vi "Destroy queues.vi"(8 "error in (no error)":errorcluster, 11 "Messenger in":refnum<class "Messenger.lvclass">) -> (0 "error out":errorcluster, 3 "Messenger out":refnum<class "Messenger.lvclass">)   [LabVIEW 2018, in "Messenger.lvclass"]
uses:
  Messenger.lvclass
  Messenger.lvclass/Messenger.ctl
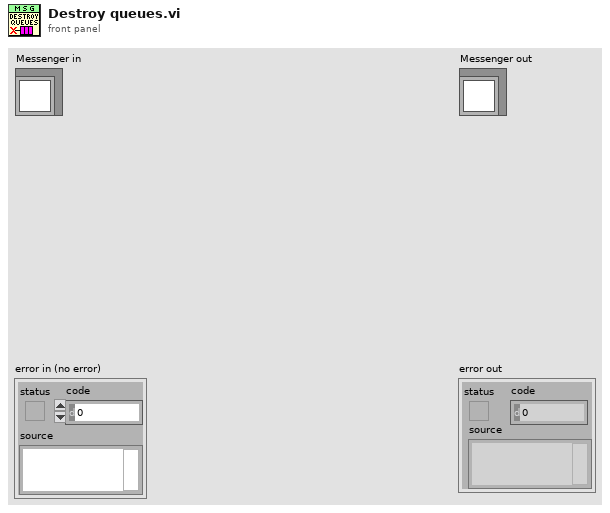
[diagram p1: front panel]
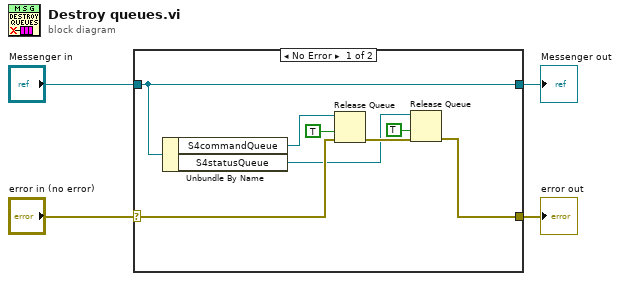
[diagram p0: block diagram]
diagram:
  n1 = case shown="No Error" "error in (no error)" {
    selector: "error in (no error)" -> [w10 w13]
    tunnel: [w9 w13] -> w3
    tunnel: [w12 w14] -> w1
    tunnel: "Messenger in" -> [w12 w14]
    frame No Error {
      n2 = Unbundle By Name(w12) -> ("S4commandQueue"=w7:refnum<queue>, "S4statusQueue"=w8:refnum<queue>)
      n3 = Release Queue(queue=w7, force destroy? (F)=TRUE, error in (no error)=w10) -> (error out=w11:errorcluster)  [unwired: 2 out]
      n4 = Release Queue(queue=w8, force destroy? (F)=TRUE, error in (no error)=w11) -> (error out=w9:errorcluster)  [unwired: 2 out]
    }
    frame Error {
    }
  }
  "error out" <- w3
  "Messenger out" <- w1
